vi "After Launch Init.vi"(8 "error in (no error)":errorcluster, 11 "CS++DMM in":refnum<class "CS++DMM.lvclass">) -> (0 "error out":errorcluster, 3 "CS++DMM out":refnum<class "CS++DMM.lvclass">)   [LabVIEW 2013, in "CS++DMM.lvlib" / "CS++DMM.lvclass"]
doc: "Use <b>Pre Launch init.vi</b> method for sanity checks that are supposed to prevent the actor from launching if they fail. Use <B>this</B> method instead to initialize this actor when it has been activated. A corresponding high priority message will become dispatched before the <B>Actor Core.vi</b> is called.\n\nRefer also to the ongoing discussion at https://decibel.ni.com/content/message/57394#57394."
uses:
  CS++DMM.lvclass
  CS++DMM.lvclass/CS++DMM.ctl
  CSPP_Core/Classes/CS++ProcessVariables/PVConnection/PVConnection.lvclass
  CSPP_Core/Actors/CS++DeviceActor/CS++DeviceActor.lvclass
  CSPP_Core/Actors/CS++DeviceActor/CS++DeviceActor.lvclass/CS++DeviceActor.ctl
  <vilib>/ActorFramework/Actor/Actor.lvclass/Actor.ctl
  <vilib>/ActorFramework/Message Enqueuer/Message Enqueuer.lvclass/Message Enqueuer.ctl
  CS++DMM Messages/Read Single-Point Msg/Read Single-Point Msg.lvclass
  CS++DMM Messages/Read Single-Point Msg/Read Single-Point Msg.lvclass/Read Single-Point Msg.ctl
  CS++DMM Messages/Read Single-Point Msg/Write maximum time.vi
  <vilib>/ActorFramework/Message Enqueuer/Init from Existing Queue.vi
  <vilib>/ActorFramework/Message Enqueuer/Message Enqueuer.lvclass
  <vilib>/ActorFramework/Actor/Actor.lvclass
  CS++DMM Messages/Read Multi-Point [MP] Msg/Read Multi-Point [MP] Msg.lvclass
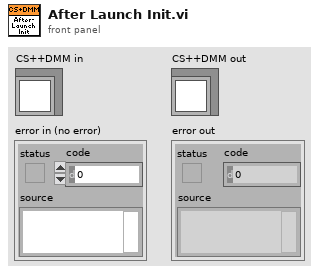
[diagram p1: front panel]
types:
  T1 = cluster{"Write Access":enum8{"Allowed", "Required", "None"}, "Read Access":enum8{"Allowed", "Required", "None"}}
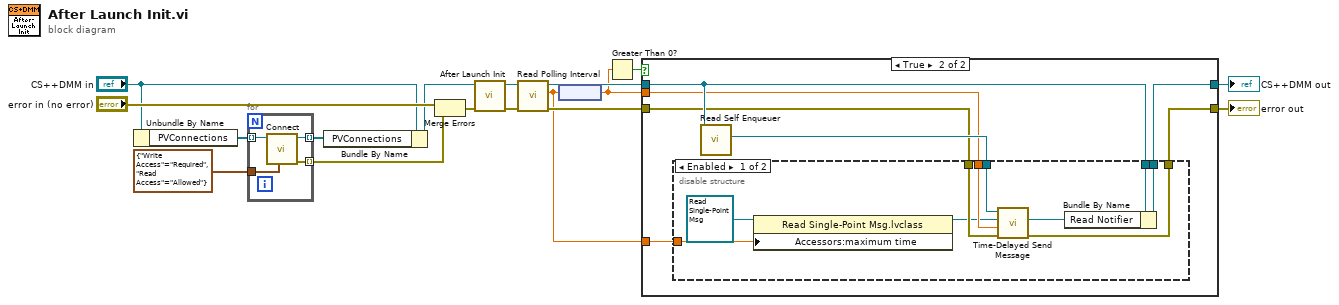
[diagram p0: block diagram]
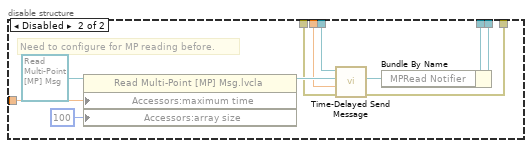
[diagram p3: hidden frame]
diagram:
  n1 = Unbundle By Name("CS++DMM in") -> ("PVConnections"=w4:refnum<class "PVConnection.lvclass">[])
  n2 = for {
    tunnel: w4 -> [w21] mode=indexing
    tunnel: [w20] -> w3 mode=indexing
    tunnel: T1 {"Write Access"=enum."Required", "Read Access"=enum."Allowed"} ("Access") -> [w19]
    tunnel: [w18] -> w2 mode=indexing
    n3 = call-dynamic "Connect.vi"("Access (R/W allowed)"=w19, "PVConnection in"=w21) -> ("error out"=w18:errorcluster, "PVConnection out"=w20:refnum<class "PVConnection.lvclass">)  [unwired: 8 in]
  }
  n4 = Bundle By Name(cluster="CS++DMM in", "PVConnections"=w3) -> (w15:refnum<class "CS++DMM.lvclass">)
  n5 = Merge Errors("error in (no error)", w2) -> (w14:errorcluster)
  n6 = call-parent "After Launch Init.vi"("error in (no error)"=w14, "CS++DeviceActor in"=w15) -> ("error out"=w9:errorcluster, "CS++DeviceActor out"=w11:refnum<class "CS++DMM.lvclass">)  [unwired: 8 in]
  n7 = call "Read Polling Interval.vi"("error in (no error)"=w9, "CS++DeviceActor in"=w11) -> ("error out"=w8:errorcluster, "Polling Interval"=w5:dbl[unit], "CS++DeviceActor out"=w10:refnum<class "CS++DMM.lvclass">)  [unwired: 7 in]
  n8 = node(w5) -> (w7:dbl)
  n9 = Greater Than 0?(x=w7) -> (x > 0?=w6:bool)
  n10 = case shown="True" w6 {
    tunnel: [w23 w30] -> w13
    tunnel: [w22 w24] -> w12
    tunnel: w10 -> [w23 w29]
    tunnel: w8 -> [w22 w27]
    tunnel: w7 -> [_ w26]
    tunnel: w5 -> [_ w25]
    frame False {
    }
    frame True {
      n11 = call <vilib>:"Read Self Enqueuer.vi"("Actor"=w29) -> ("Self Enqueuer"=w28:refnum<class "Message Enqueuer.lvclass">)  [unwired: 10 in]
      n12 = disable-structure shown="Enabled" {
        disable-tunnel: [w40 w43] -> w30
        disable-tunnel: w29 -> [w39 w44]
        disable-tunnel: w28 -> [w37 w47]
        disable-tunnel: w27 -> [w36 w45]
        disable-tunnel: w26 -> [w35 w46]
        disable-tunnel: w25 -> [w32 w48]
        disable-tunnel: [w31 w41] -> w24
        frame Enabled {
          n13 = property class="Read Single-Point Msg.lvclass"(reference=refnum<class "Read Single-Point Msg.lvclass"> refnum ("CS++DMM.lvlib:Read Single-Point Msg.lvclass"), "Accessors:maximum time"=w32) -> (reference out=w33:refnum<class "Read Single-Point Msg.lvclass">)  [unwired: 1 in, 1 out]
          n14 = call <vilib>:"Time-Delayed Send Message.vi"("error in (no error)"=w36, "Milliseconds To Wait"=w35, "Message"=w33, "Message Enqueuer"=w37) -> ("error out"=w31:errorcluster, "Delivery Notifier"=w38:refnum<notifier>)  [unwired: 6 in]
          n15 = Bundle By Name(cluster=w39, "Read Notifier"=w38) -> (w40:refnum<class "CS++DMM.lvclass">)
        }
        frame Disabled {
          # "Need to configure for MP reading before."
          n16 = property class="Read Multi-Point [MP] Msg.lvcla"(reference=refnum<class "Read Multi-Point [MP] Msg.lvclass"> refnum ("CS++DMM.lvlib:Read Multi-Point [MP] Msg.lvclass"), "Accessors:maximum time"=w48, "Accessors:array size"=100 ("array size")) -> (reference out=w50:refnum<class "Read Multi-Point [MP] Msg.lvclass">)  [unwired: 1 in, 1 out]
          n17 = call <vilib>:"Time-Delayed Send Message.vi"("error in (no error)"=w45, "Milliseconds To Wait"=w46, "Message"=w50, "Message Enqueuer"=w47) -> ("error out"=w41:errorcluster, "Delivery Notifier"=w42:refnum<notifier>)  [unwired: 6 in]
          n18 = Bundle By Name(cluster=w44, "MPRead Notifier"=w42) -> (w43:refnum<class "CS++DMM.lvclass">)
        }
      }
    }
  }
  "error out" <- w12
  "CS++DMM out" <- w13
